vi "StatusUpdate Callback.vi"(4 "Inertial Motor Status":refnum<user-event>, 5 "Event Data":cluster{"sender":refnum<k24>, "e":refnum<k24>}, 6 "Control Ref":refnum<k24>, 7 "Event Common Data":T1) -> ()   [LabVIEW 2017, in "XYStage.KIM101.lvclass"]
uses:
  XYStage.KIM101.lvclass
  D:/upwork/Laser Measurement Tool/Laser/project/data/Thorlabs.MotionControl.KCube.InertialMotorCLI.dll
  data/Thorlabs.MotionControl.KCube.InertialMotorCLI.dll
  Typedefs/InertialMotorStatus--Cluster.ctl
panel:
  out "error out":errorcluster
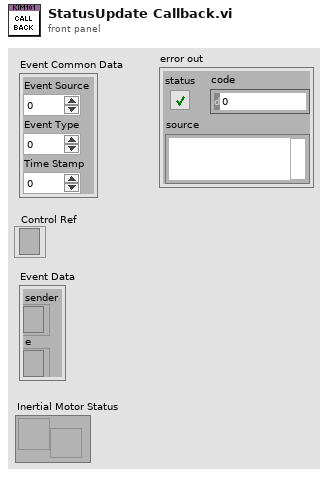
[diagram p1: front panel]
types:
  T1 = cluster{"Event Source":i32, "Event Type":u32, "Time Stamp":u32}
  T2 = typedef "XYStage.KIM101.lvclass/InertialMotorStatus--Cluster.ctl" = cluster{"Channel":i32, "IsEnabled":bool, "IsError":bool, "IsMoving":bool, "Position":i32, "Status":u32}
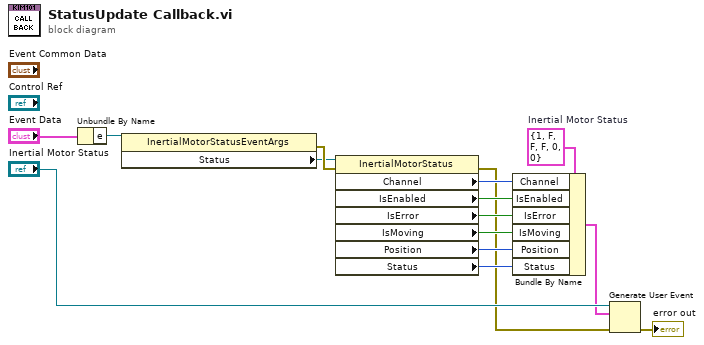
[diagram p0: block diagram]
diagram:
  w11 = T2 {"Channel"=1, "IsEnabled"=FALSE, "IsError"=FALSE, "IsMoving"=FALSE, "Position"=0, "Status"=0}  # Inertial Motor Status
  n1 = Unbundle By Name("Event Data") -> ("e"=w14:refnum<k24>)
  n2 = property class="InertialMotorStatusEventArgs"(reference=w14) -> (error out=w13:errorcluster, "Status"=w12:refnum<k24>)  [unwired: 1 in, 1 out]
  n3 = property class="InertialMotorStatus"(reference=w12, error in=w13) -> (error out=w2:errorcluster, "Channel"=w10:i32, "IsEnabled"=w9:bool, "IsError"=w8:bool, "IsMoving"=w7:bool, "Position"=w6:i32, "Status"=w5:u32)  [unwired: 1 out]
  n4 = Bundle By Name(cluster=w11, "Channel"=w10, "IsEnabled"=w9, "IsError"=w8, "IsMoving"=w7, "Position"=w6, "Status"=w5) -> (w3:T2)
  n5 = Generate User Event(user event="Inertial Motor Status", event data cluster=w3, error in=w2) -> (error out=→"error out":errorcluster)  [unwired: 1 in, 1 out]
